vi "S2C_Shared_Proc_ClearLog.vi"(8 "Error In":errorcluster, 11 "Refs":string[][](array[string])) -> (0 "Error Out":errorcluster)   [LabVIEW 2024]
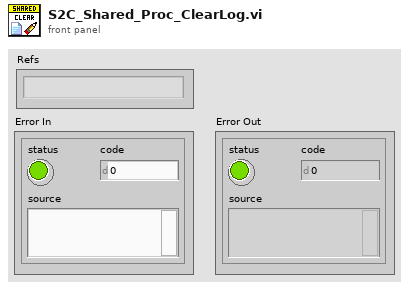
[diagram p1: front panel]
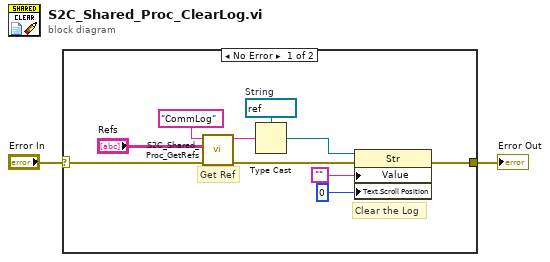
[diagram p0: block diagram]
diagram:
  n1 = case shown="No Error" "Error In" {
    selector: "Error In" -> [w5 w13]
    tunnel: [w3 w13] -> w1
    frame No Error {
      w12 = refnum<vi> refnum  # String
      # "Clear the Log"
      # "Get Ref"
      n2 = call "S2C_Shared_Proc_GetRefs.vi"("Error In"=w5, "Refs"="Refs", "Label"="CommLog") -> ("Error Out"=w9:errorcluster, "Reference"=w11:string)  [unwired: 7 in]
      n3 = Type Cast(type=w12, x=w11) -> (*(type *) &x=w6:refnum<vi>)
      n4 = property on="Property Node" class="Str"(reference=w6, error in=w9, "Value"="", "Text.Scroll Position"=u32 0) -> (error out=w3:errorcluster)  [unwired: 1 out]
    }
    frame Error {
    }
  }
  "Error Out" <- w1
